vi "CoinDetection_new.vi"(0 "Min Radius (Circle Detection 1)":sgl=3.0, 1 "Max Radius (Circle Detection 1)":sgl=100.0, 7 "error in":errorcluster) -> (20 "Nb Circles (Circle Detection 1)":i32, 21 "Circles Data (Circle Detection 1)":T2(array[cluster]), 22 "Circles Data (calibrated) (Circle Detection 1)":T2(array[cluster]), 27 "error out":errorcluster)   [LabVIEW 2015]
uses:
  <vilib>/vision/NI_Vision_Development_Module.lvlib
panel:
  out "Image Out":T1(plugin-control)
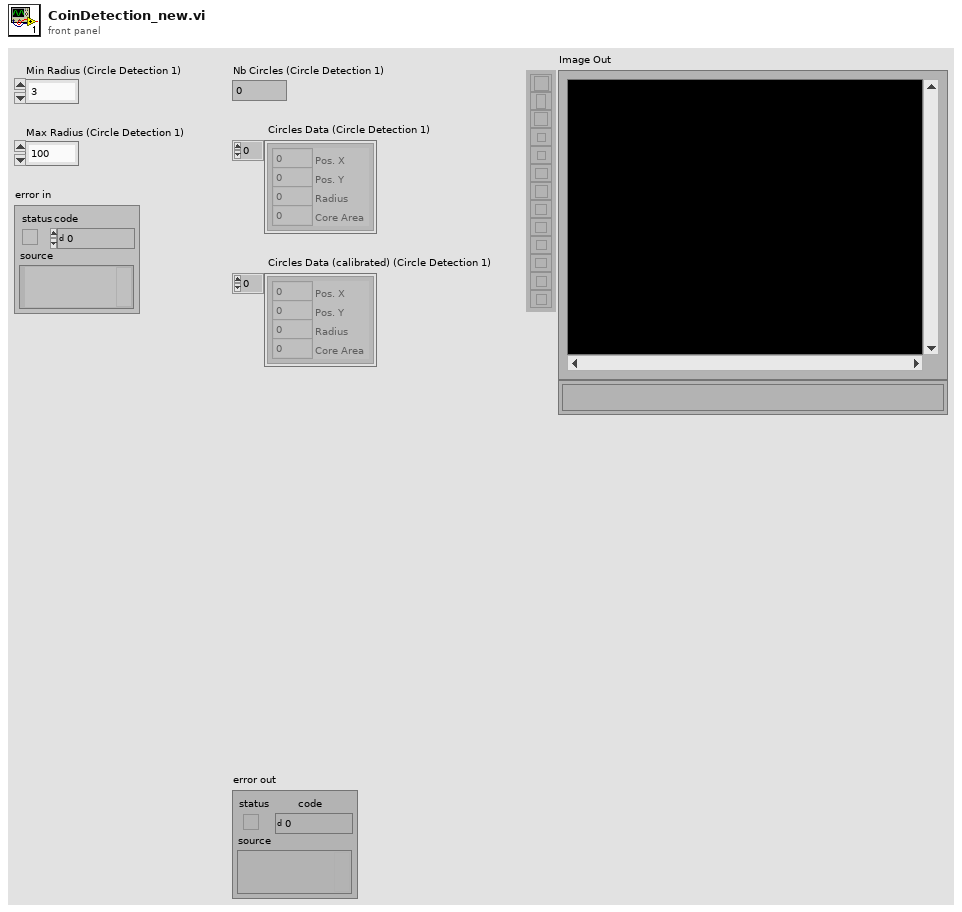
[diagram p1: front panel]
types:
  T1 = typedef "IMAQ Image.ctl" = refnum<image>
  T2 = cluster{"Pos. X":i32, "Pos. Y":i32, "Radius":i32, "Core Area":i32}[]
  T3 = enum32{"AutoM", "Close", "Dilate", "Erode", "Gradient", "Gradient out", "Gradient in", "Hit miss", "Open", "PClose", "POpen", "Thick", "Thin"}
  T4 = typedef "Image Type" = u32
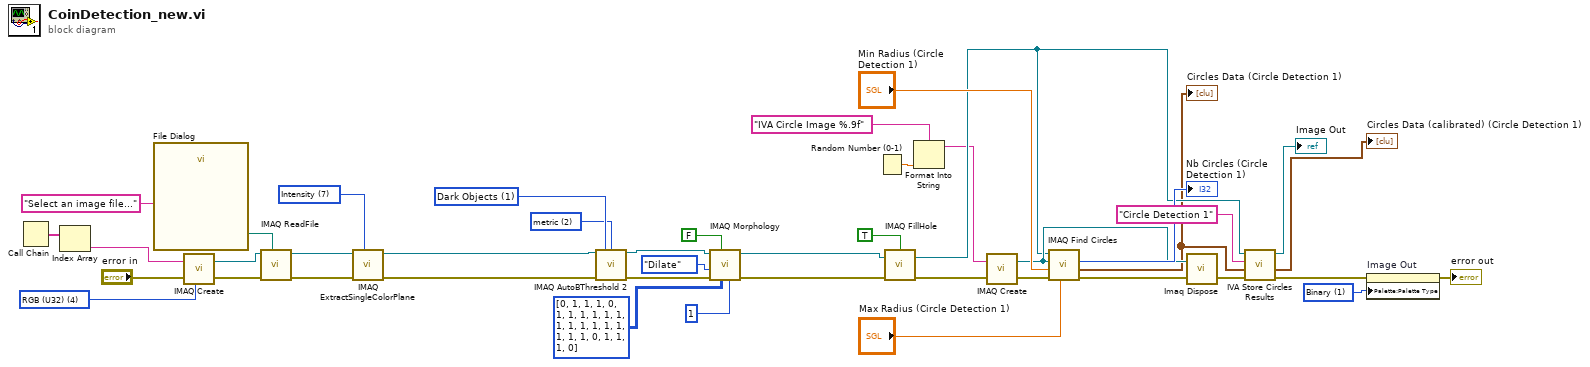
[diagram p0: block diagram]
diagram:
  w1 = u32 1 items=["Grayscale", "Binary", "Gradient", "Rainbow", "Temperature", "User Defined", "Binary 16 Bit", "Gradient 16 Bit", "Rainbow 16 Bit", "Temperature 16 Bit", "User Defined 16 Bit"] ("Palette Type")
  w29 = 2 items=["clustering", "entropy", "metric", "moments", "inter-class variance"] ("Method")
  w30 = u32 1 items=["Bright Objects", "Dark Objects"] ("Look For")
  w35 = 7 items=["Red", "Green", "Blue", "Hue", "Saturation", "Luminance", "Value", "Intensity"] ("Color Plane")
  w36 = T4 4 items=["Grayscale (U8)", "Grayscale (I16)", "Grayscale (SGL)", "Complex (CSG)", "RGB (U32)", "HSL (U32)", "RGB (U64)", "Grayscale (U16)"] ("Image Type")
  n1 = Call Chain() -> (call chain=w40:string[])
  n2 = Index Array(array=w40) -> (element=w39:string)  [unwired: 1 in]
  n3 = call "File Dialog"("prompt"="Select an image file...") -> ("selected path"=w37:path)  [unwired: 6 in, 8 out]
  n4 = call "IMAQ Create"("Image Name"=w39, "Image Type"=w36, "error in (no error)"="error in") -> ("New Image"=w43:T1, "error out"=w42:errorcluster)  [unwired: 1 in, 1 out]
  n5 = call "IMAQ ReadFile"("File Path"=w37, "error in (no error)"=w42, "Image"=w43) -> ("error out"=w33:errorcluster, "Image Out"=w34:T1)  [unwired: 2 in, 5 out]
  n6 = call "IMAQ ExtractSingleColorPlane"("Color Plane"=w35, "error in (no error)"=w33, "Image Src"=w34) -> ("error out"=w32:errorcluster, "Image Dst Out"=w31:T1)  [unwired: 1 in, 6 out]
  n7 = call "IMAQ AutoBThreshold 2"("Image Src"=w31, "Look For (Bright Objects)"=w30, "Method (clustering)"=w29, "error in (no error)"=w32) -> ("Image Dst Out"=w24:T1, "error out"=w23:errorcluster)  [unwired: 4 in, 6 out]
  n8 = call "IMAQ Morphology"("Number of iterations (1)"=1, "Structuring Element"=i32[][] [[0, 1, 1, 1, 0], [1, 1, 1, 1, 1], [1, 1, 1, 1, 1], [1, 1, 1, 1, 1], [0, 1, 1, 1, 0]], "Square/Hexa (Square)"=FALSE, "error in (no error)"=w23, "Operation"=T3."Dilate", "Image Src"=w24) -> ("error out"=w20:errorcluster, "Image Dst Out"=w21:T1)  [unwired: 1 in, 3 out]
  n9 = Random Number (0-1)() -> (number: 0 to 1=w5:dbl)
  n10 = call "IMAQ FillHole"("error in (no error)"=w20, "Image Src"=w21, "Connectivity 4/8 (8)"=TRUE) -> ("error out"=w14:errorcluster, "Image Dst Out"=w11:T1)  [unwired: 1 in, 2 out]
  n11 = Format Into String(format string="IVA Circle Image %.9f" ("Image Name"), w5) -> (resulting string=w7:string)  [unwired: 2 in, 1 out]
  n12 = call "IMAQ Create"("Image Name"=w7, "error in (no error)"=w14) -> ("New Image"=w16:T1, "error out"=w15:errorcluster)  [unwired: 2 in, 1 out]
  n13 = call "IMAQ Find Circles"("Max Radius"="Max Radius (Circle Detection 1)", "error in (no error)"=w15, "Min Radius"="Min Radius (Circle Detection 1)", "Image Dst"=w16, "Image Src"=w11) -> ("error out"=w13:errorcluster, "Circles Data"=w9:T2, "Nb Circles"=→"Nb Circles (Circle Detection 1)":i32)  [unwired: 4 out]
  "Circles Data (Circle Detection 1)" <- w9
  n14 = call "Imaq Dispose"("Image"=w16, "error in (no error)"=w13) -> ("error out"=w12:errorcluster)  [unwired: 1 in, 3 out]
  n15 = call <vilib>:"IVA Store Circles Results.vi"("error in (no error)"=w12, "Circles Data"=w9, "Step Name"="Circle Detection 1", "Image in"=w11) -> ("error out"=w4:errorcluster, "Circles Data (calibrated)"=→"Circles Data (calibrated) (Circle Detection 1)":T2, "Image dup"=→"Image Out":T1)  [unwired: 5 out]
  n16 = property on="Image Out" class="ImageControl"(error in=w4, "Palette:Palette Type"=w1) -> (error out=→"error out":errorcluster)  [unwired: 1 in, 1 out]
